vi "NI_FPGA_PPG.start.vi"(0 "i ref in":refnum<vi>, 2 "start_addr":i32, 3 "ms timeout (10000)":i32=10000, 5 "error in (no error)":errorcluster, 7 "ignorePdcHandling":bool) -> (14 "i ref out":refnum<vi>, 17 "timed out":bool, 19 "error out":errorcluster)   [LabVIEW 2014, in "NI_FPGA_PPG.lvlib"]
doc: "Starts the execution of the pattern generation on the FPGA target.\n\nLicense Agreement for this software:\n\nCopyright (C) 2009\nFalk Ziegler\nInstitut für Physik\nErnst-Moritz-Arndt Universität\nFelix-Hausdorff-Str. 6\n17487 Greifswald\n\nContact: Falk Ziegler, ziegler@physik.uni-greifswald.de\n\nThis program is free software: you can redistribute it and/or modify it under the terms of the GNU General Public License as published by the Free Software Foundation, either version 3 of the License, or (at your option) any later version.\n\nThis program is distributed in the hope that it will be useful, but WITHOUT ANY WARRANTY; without even the implied warranty of MERCHANTABILITY or FITNESS FOR A PARTICULAR PURPOSE. See the GNU General Public License for more details.\n\nYou should have received a copy of the GNU General Public License along with this program. If not, see <http://www.gnu.org/licenses/>.\n\nFor all questions and ideas contact: ziegler@physik.uni-greifswald.de or d.beck@gsi.de\nLast update: 01-Sep-2009"
uses:
  NI_FPGA_PPG.lvlib
  CSCore/CSApplicationBaseClasses/DeviceBase/DeviceBase.lvlib
  CSinstr.lib/NI-FPGA-PPG/host/instrumentDriver/NI-FPGA_PPG_Driver.lvlib
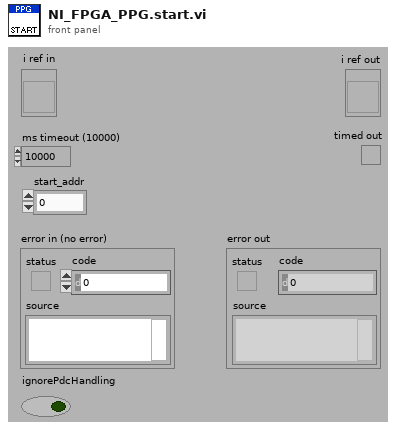
[diagram p1: front panel]
types:
  T1 = typedef "NI_FPGA_PPG.lvlib/NI_FPGA_PPG.i attribute.ctl" = cluster{"dim_service_id":cluster{"dim_actual_device_status":i32, "dim_event_data":i32, "dim_cmd_data":i32, "dim_cmd_data _description":i32, "dim_channel_description":i32}, "VISA":refnum<visa-resource-name>, "actual_device_status":i32, "event_data_id":i32, "pdc_enabled":bool, "pdc_timestamp":u32, "cmd_data_string":string, "cmd_data_size":i32, "cmd_data_description_string":string, "cmd_data_description_size":i32, "channel_description_string":string, "channel_description_size":i32}
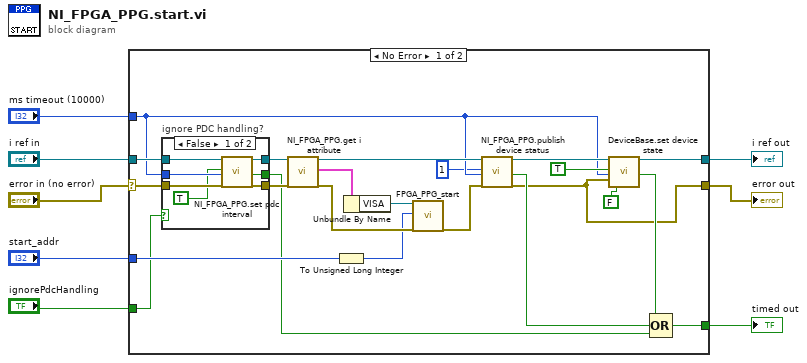
[diagram p0: block diagram]
diagram:
  n1 = case shown="No Error" "error in (no error)" {
    selector: "error in (no error)" -> [w19 w41]
    tunnel: "i ref in" -> [w20 w42]
    tunnel: [w27 w42] -> w6
    tunnel: [w13 w41] -> w5
    tunnel: "ms timeout (10000)" -> [w16 _]
    tunnel: "start_addr" -> [w28 _]
    tunnel: [w24 _] -> w2
    tunnel: "ignorePdcHandling" -> [w9 _]
    frame No Error {
      n2 = case "ignore PDC handling?" shown="False" w9 {
        tunnel: [w38 w40] -> w22
        tunnel: [w37 w39] -> w21
        tunnel: w20 -> [w36 w40]
        tunnel: w19 -> [w35 w39]
        tunnel: w16 -> [w34 _]
        tunnel: [w33 _] -> w15
        frame False {
          n3 = call "NI_FPGA_PPG.set pdc interval.vi"("i ref in"=w36, "enable_pdc"=TRUE, "ms timeout (10000)"=w34, "error in (no error)"=w35) -> ("i ref out"=w38:refnum<vi>, "timed out"=w33:bool, "error out"=w37:errorcluster)  [unwired: 13 in]
        }
        frame True {
        }
      }
      n4 = call "NI_FPGA_PPG.get i attribute.vi"("i ref in"=w22, "error in (no error)"=w21) -> ("i ref out"=w18:refnum<vi>, "i attribute"=w31:T1, "error out"=w29:errorcluster)  [unwired: 15 in]
      n5 = To Unsigned Long Integer(number=w28) -> (unsigned 32bit integer=w12:u32)
      n6 = Unbundle By Name(w31) -> ("VISA"=w30:refnum<visa-resource-name>)
      n7 = call "FPGA_PPG_start.vi"("resource_in"=w30, "start_addr"=w12, "error in (no error)"=w29) -> ("error out"=w11:errorcluster)  [unwired: 15 in, 1 out]
      n8 = call "NI_FPGA_PPG.publish device status.vi"("i ref in"=w18, "actual_status"=1, "ms timeout (10000)"=w16, "error in (no error)"=w11) -> ("i ref out"=w17:refnum<vi>, "timed out"=w14:bool, "error out"=w13:errorcluster)  [unwired: 13 in]
      n9 = call "DeviceBase.set device state.vi"("i ref in"=w17, "implicit"=TRUE, "ms timeout (10000)"=w16, "device error"=w13, "mayResetError (FALSE)"=FALSE) -> ("i ref out"=w27:refnum<vi>, "timed out"=w23:bool)  [unwired: 12 in, 1 out]
      n10 = Compound Arithmetic op=OR(w23, w14, w15) -> (w24:bool)
    }
    frame Error {
    }
  }
  "error out" <- w5
  "i ref out" <- w6
  "timed out" <- w2
